vi "Keithley J-t List_IIT.vi"(0 "VISA resource name in":refnum<visa-resource-name>, 1 "Shutter open?":bool, 7 "t=0 timestamp":sgl, 9 "Light?":bool, 11 "error in (no error)":errorcluster, 12 "Voltage List":dbl[](array[numeric])) -> (4 "VISA resource name out":refnum<visa-resource-name>, 6 "Data Array":dbl[][](array[numeric]), 8 "timestamp":sgl, 15 "Measurement Complete":bool)   [LabVIEW 2016]
doc: "Configures a sweep and takes voltage and current readings at each point."
uses:
  C:/Program Files (x86)/National Instruments/LabVIEW 2016/instr.lib/keithley_24xx/Keithley 24XX/Public/Data/Read (Multiple Points).vi
  C:/Program Files (x86)/National Instruments/LabVIEW 2016/instr.lib/keithley_24xx/Keithley 24XX/Keithley 24XX.lvlib
panel:
  in  "Source Mode  (0: Voltage)":u16(ring) items=["Voltage", "Current"]
  # "(c) 2006 National Instruments.  ALL RIGHTS RESERVED."
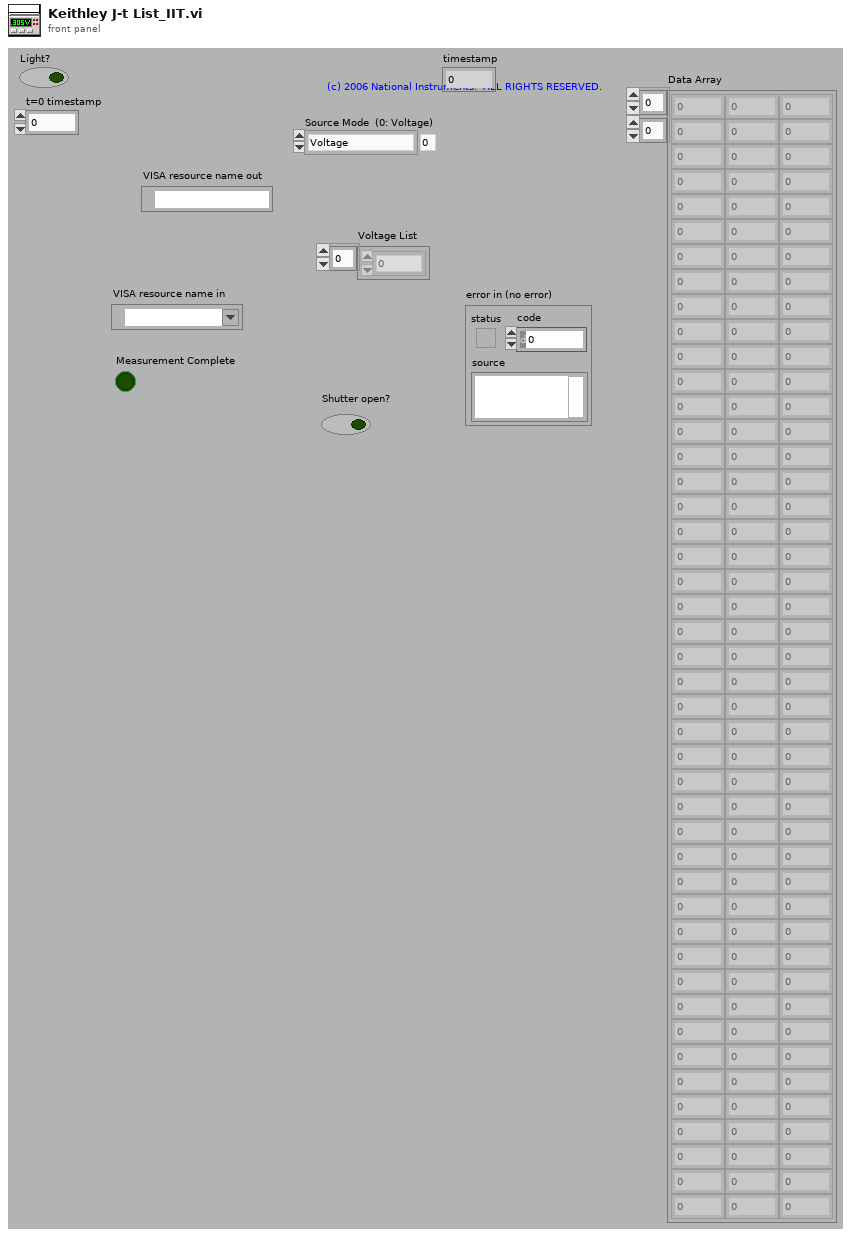
[diagram p1: front panel]
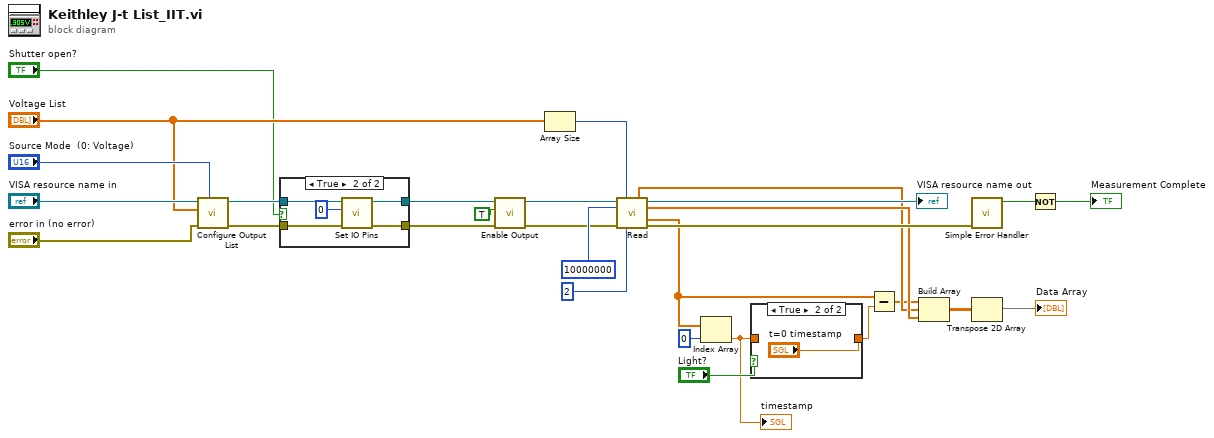
[diagram p0: block diagram]
diagram:
  n1 = call "Configure Output List.vi"("Source Mode  (0: Voltage)"="Source Mode  (0: Voltage)", "error in (no error)"="error in (no error)", "Output List"="Voltage List", "VISA resource name"="VISA resource name in") -> ("error out"=w7:errorcluster, "VISA resource name out"=w8:refnum<visa-resource-name>)  [unwired: 6 in]
  n2 = case shown="True" "Shutter open?" {
    tunnel: w8 -> [w31 w35]
    tunnel: w7 -> [w30 w34]
    tunnel: [w31 w33] -> w6
    tunnel: [w30 w32] -> w5
    frame False {
    }
    frame True {
      n3 = call "Set IO Pins.vi"("error in (no error)"=w34, "Output Pattern (0)"=0, "VISA resource name"=w35) -> ("error out"=w32:errorcluster, "VISA resource name out"=w33:refnum<visa-resource-name>)  [unwired: 7 in]
    }
  }
  n4 = call "Enable Output.vi"("error in (no error)"=w5, "Enable Output (T: Enable)"=TRUE ("Output (Off)"), "VISA resource name"=w6) -> ("error out"=w3:errorcluster, "VISA resource name out"=w4:refnum<visa-resource-name>)  [unwired: 7 in]
  n5 = Array Size(array="Voltage List") -> (size(s)=w19:i32)
  n6 = call-poly "Read.vi"("VISA resource name"=w4, "Sample Count (1)"=w19, "Timeout (10000 ms)"=10000000, "error in (no error)"=w3, "Output Mode (0: Fixed)"=2) -> ("Voltage"=w18:sgl[], "VISA resource name out"=→"VISA resource name out":refnum<visa-resource-name>, "Current"=w21:sgl[], "Timestamp"=w16:sgl[], "error out"=w29:errorcluster)  [unwired: 4 in, 2 out]
  n7 = Index Array(array=w16, index=0) -> (element=w12:sgl)
  "timestamp" <- w12
  n8 = case shown="True" "Light?" {
    tunnel: [w37 "t=0 timestamp"] -> w13
    tunnel: w12 -> [w37 _]
    frame False {
    }
    frame True {
    }
  }
  n9 = Subtract(x=w16, y=w13) -> (x-y=w17:sgl[])
  n10 = Build Array(w17, w18, w21) -> (w11:sgl[][])
  n11 = call <vilib>:"Simple Error Handler.vi"("error in (no error)"=w29) -> ("error?"=w27:bool)  [unwired: 4 in, 4 out]
  n12 = Transpose 2D Array(2D array=w11) -> (transposed array=→"Data Array":sgl[][])
  n13 = Not(x=w27) -> (.not. x?=→"Measurement Complete":bool)
